vi "Report Error.vi"(8 "error in (no error)":errorcluster, 9 "Message":string, 10 "Context":string, 11 "Event API in":refnum<class "EventAPI.lvclass">) -> (0 "error out":errorcluster, 3 "Event API out":refnum<class "EventAPI.lvclass">)   [LabVIEW 2020, in "Volatus.lvlib" / "EventAPI.lvclass"]
uses:
  EventAPI.lvclass
  Event Level.ctl
  EventAPI.lvclass/EventAPI.ctl
  EventHandler Messages/Handle Event Msg/Handle Event Msg.lvclass/Handle Event Msg.ctl
  <vilib>/ActorFramework/Message Enqueuer/Message Enqueuer.lvclass/Message Enqueuer.ctl
  EventHandler Messages/Handle Event Msg/Send Handle Event.vi
  <vilib>/ActorFramework/Message Enqueuer/Enqueue.vi
  EventHandler Messages/Handle Event Msg/Handle Event Msg.lvclass
  C:/Program Files (x86)/National Instruments/LabVIEW 2020/vi.lib/ActorFramework/Message/Message.lvclass
  <vilib>/ActorFramework/Message Priority Queue/Priority Enqueue.vi
  Volatus.lvlib
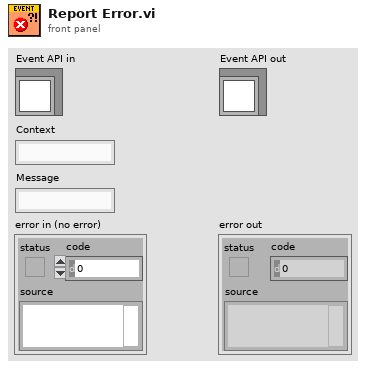
[diagram p1: front panel]
types:
  T1 = typedef "Volatus.lvlib/Event Level.ctl" = enum16{"Debug", "Info", "Warning", "Error"}
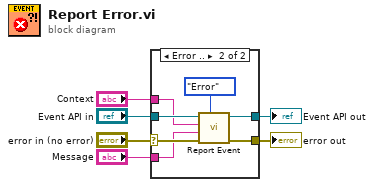
[diagram p0: block diagram]
diagram:
  n1 = case shown="Error .." "error in (no error)" {
    selector: "error in (no error)" -> [w8 w15]
    tunnel: "Event API in" -> [w7 w13]
    tunnel: "Context" -> [_ w12]
    tunnel: [w8 w11] -> w3
    tunnel: [w7 w10] -> w2
    tunnel: "Message" -> [_ w9]
    frame No Error {
    }
    frame Error {
      n2 = call "Report Event.vi"("Level (Info)"=Event_Level."Error", "error in (no error)"=w15, "Message"=w9, "Context"=w12, "Event API in"=w13) -> ("error out"=w11:errorcluster, "Event API out"=w10:refnum<class "EventAPI.lvclass">)  [unwired: 5 in]
    }
  }
  "error out" <- w3
  "Event API out" <- w2
